vi "Read_Temperature.vi"(0 "error in":errorcluster) -> (1 "error out":errorcluster, 2 "Termperature":dbl)   [LabVIEW 2010]
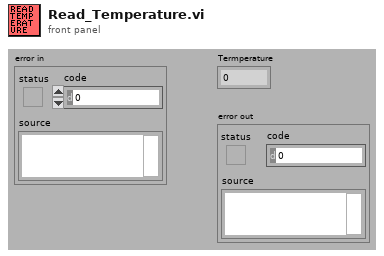
[diagram p1: front panel]
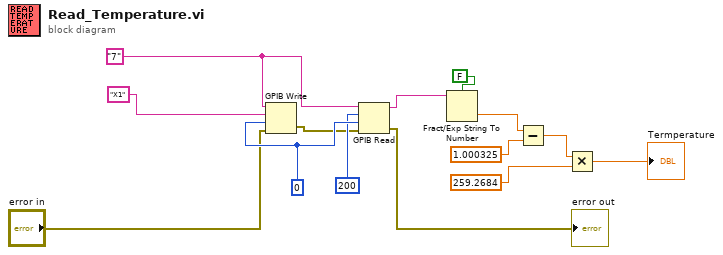
[diagram p0: block diagram]
diagram:
  w10 = 0
  w11 = "7"
  n1 = GPIB Write(0:w11, 1:"X1", 2:w10, 3:"error in") -> (6:w8:errorcluster)  [unwired: 1 in, 1 out]
  n2 = GPIB Read(0:w11, 1:200, 2:w10, 3:w8) -> (5:w13:string, 7:→"error out":errorcluster)  [unwired: 1 in, 1 out]
  n3 = Fract/Exp String To Number(use system decimal point (T)=FALSE, string=w13) -> (number=w4:dbl)  [unwired: 2 in, 1 out]
  n4 = Subtract(x=w4, y=1.000325) -> (x-y=w2:dbl)
  n5 = Multiply(x=w2, y=259.2684) -> (x*y=→"Termperature":dbl)
